vi "IX81 Device Engine.vi"(0 "Unique Notifier Name":string, 11 "COM Port":string[](array[string])) -> ()   [LabVIEW 2020]
uses:
  Microscopes Type Defs/Microscope Notifier.ctl
  Microscopes Type Defs/Microscope Actions.ctl
  <vilib>/Instr/_visa.llb/VISA Configure Serial Port (Instr).vi
panel:
  out "Objective Z Position (um)":dbl
  in  "Lock Base":bool
  out "Last Error":errorcluster
  in  "Quit":bool
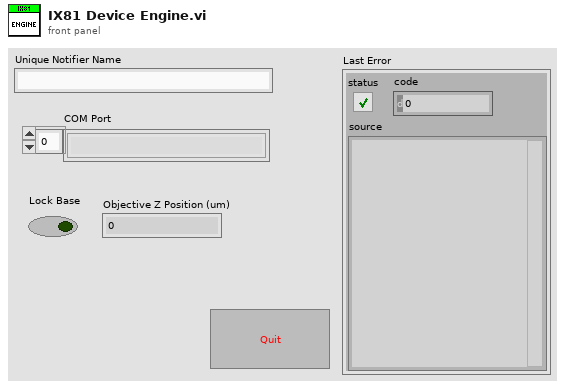
[diagram p1: front panel]
types:
  T1 = typedef "Microscope Actions.ctl" = enum16{"Do Nothing", "Lock Base", "Get Objective Index", "Get Objective Z Position", "Get Lamp State", "Get Lamp Power", "Get Output Port", "Get Shutter State", "Get Dichroic Wheel Position", "Set Lamp Index", "Set Shutter Index", "Set Objective Z Position", "Set Lamp State", "Set Lamp Power", "Set Output Port", "Set Shutter State", "Set Dichroic Wheel Position", "Set Objective", "Abort Move", "Set Parameter", "Get Parameter", "Quit"}
  T2 = typedef "Microscope Notifier.ctl" = cluster{"Actions":T1, "Action Done":bool, "Objective Index":u8, "Objective Z Position (um)":dbl, "Lamp Index":u8, "Lamp State":bool, "Output Port":u8, "Shutter Index":u8, "Shutter State":bool, "Dichroic Wheel Position":u8, "Parameter":string, "Parameter Value":string, "Base Locked?":bool, "Obj Speed":u32, "Obj Acceleration":u32, "Obj Deceleration":u32, "Lamp Power (%)":dbl}
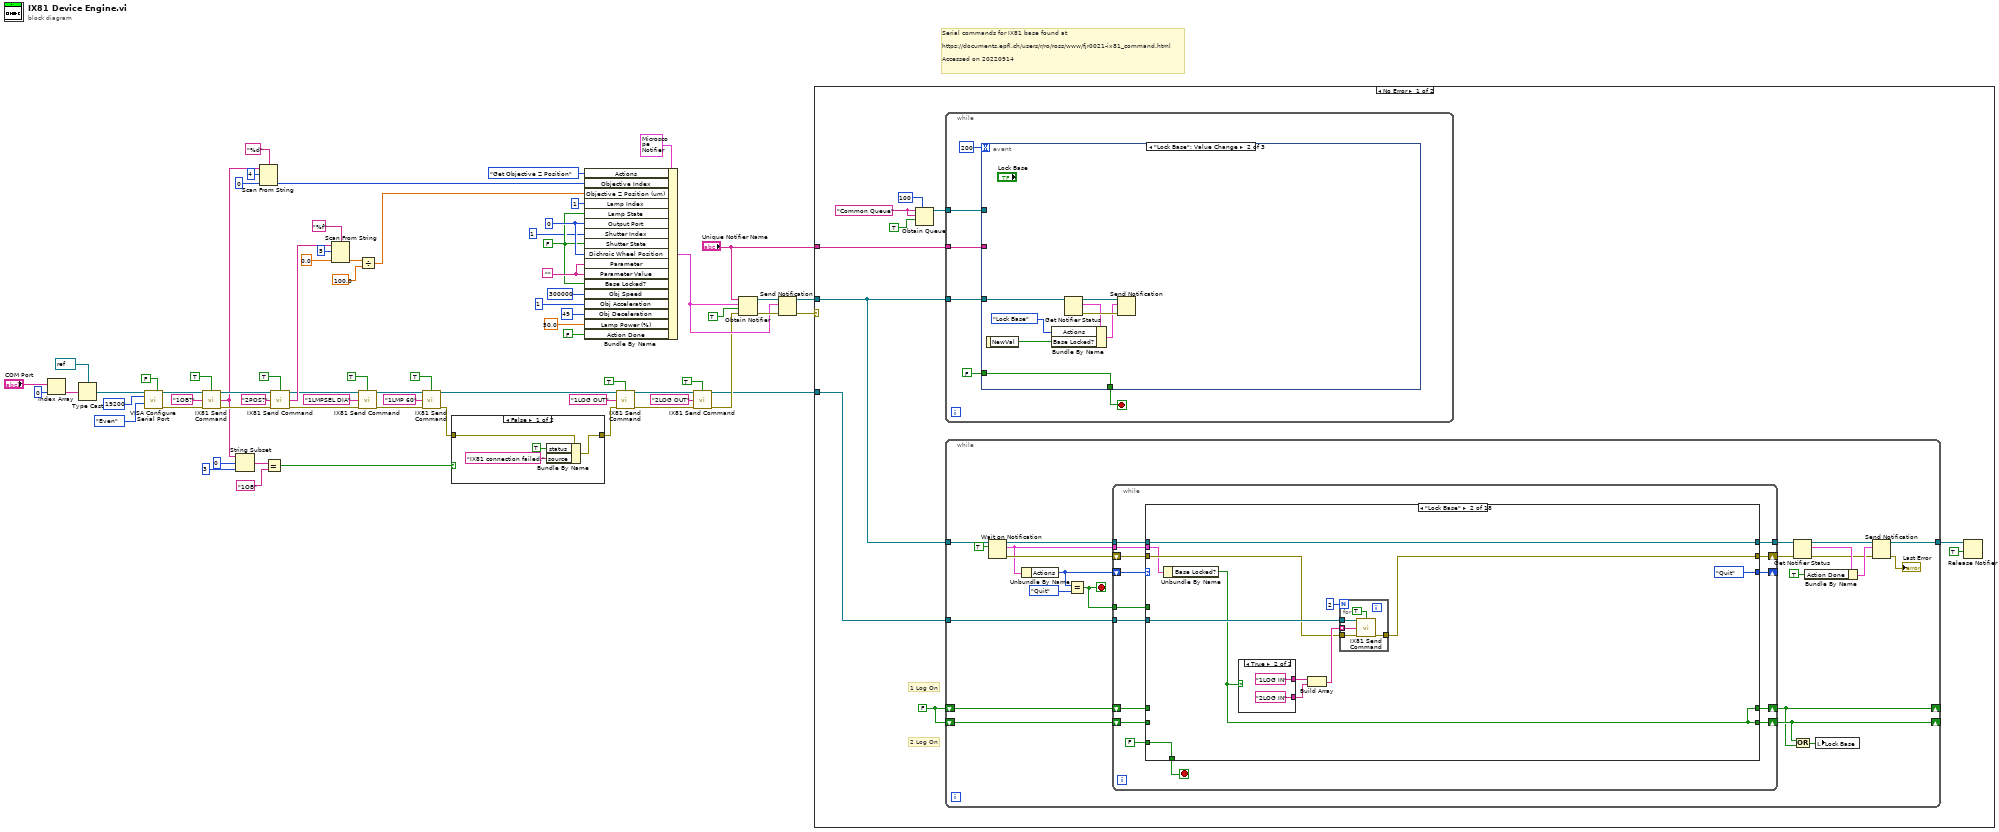
[diagram p0: block diagram]
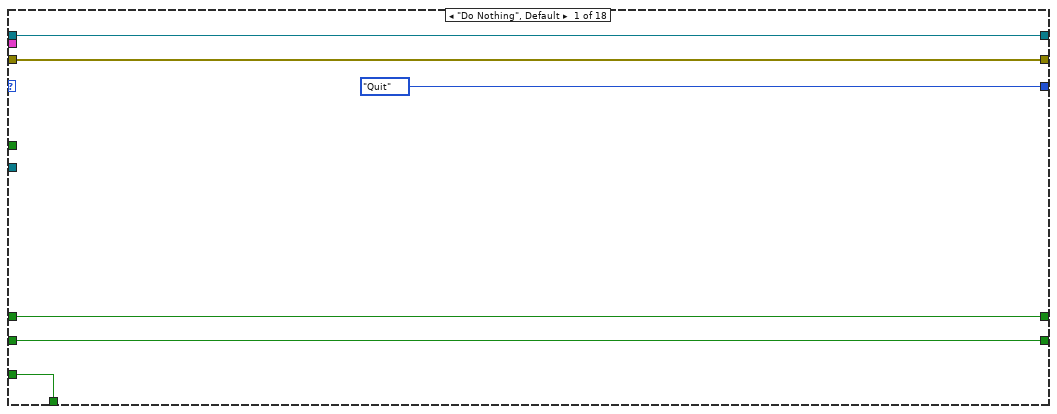
[diagram p2: hidden frame]
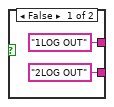
[diagram p3: hidden frame]
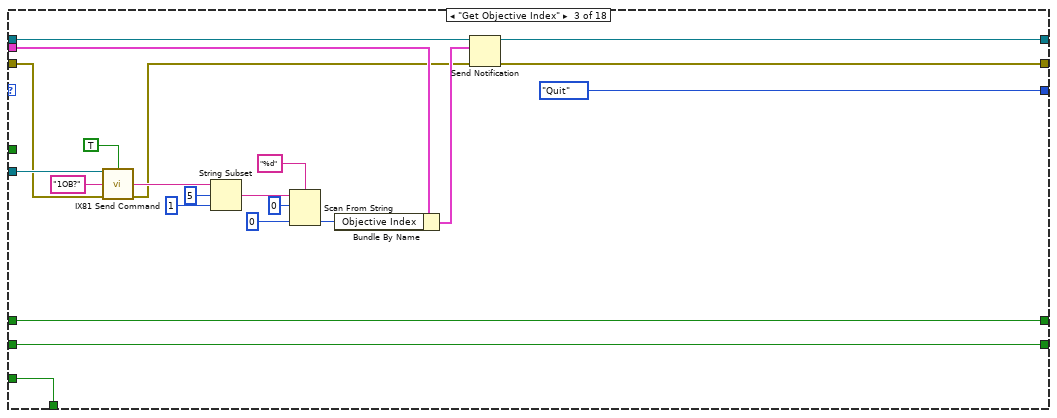
[diagram p4: hidden frame]
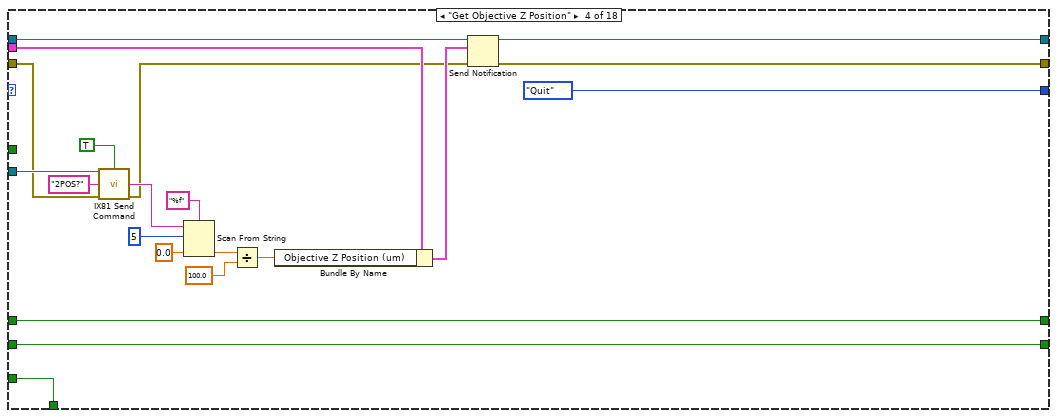
[diagram p5: hidden frame]
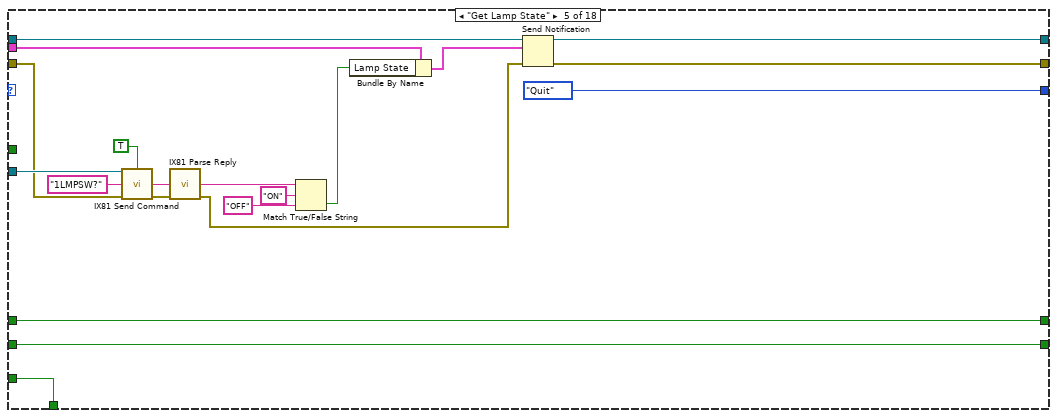
[diagram p6: hidden frame]
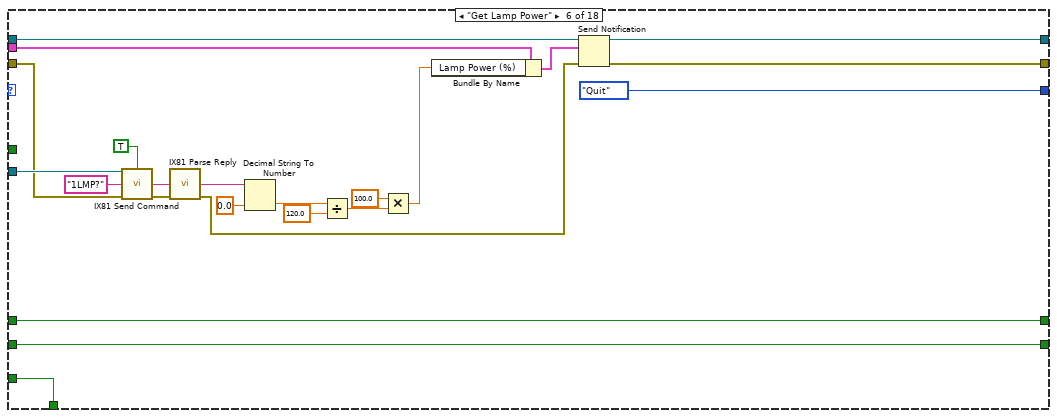
[diagram p7: hidden frame]
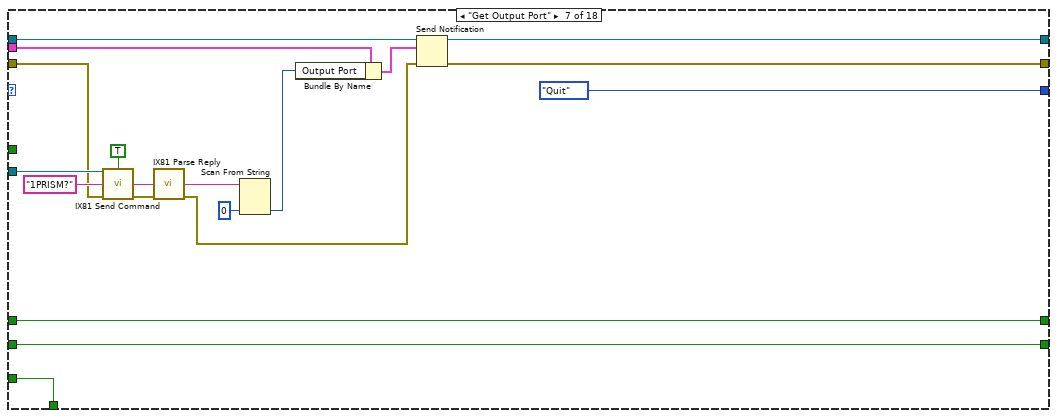
[diagram p8: hidden frame]
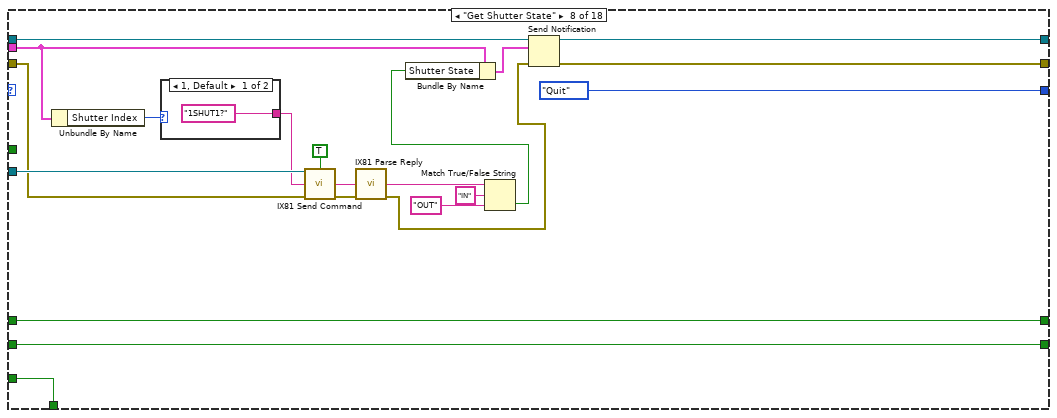
[diagram p9: hidden frame]
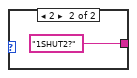
[diagram p10: hidden frame]
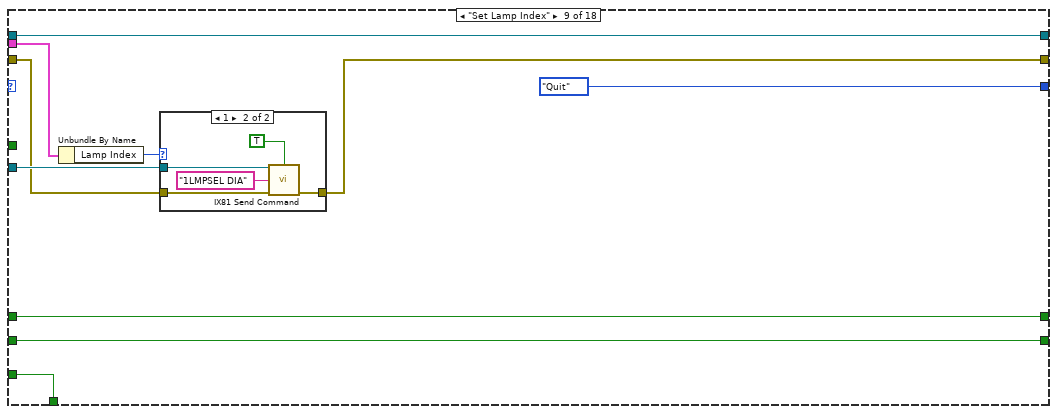
[diagram p11: hidden frame]
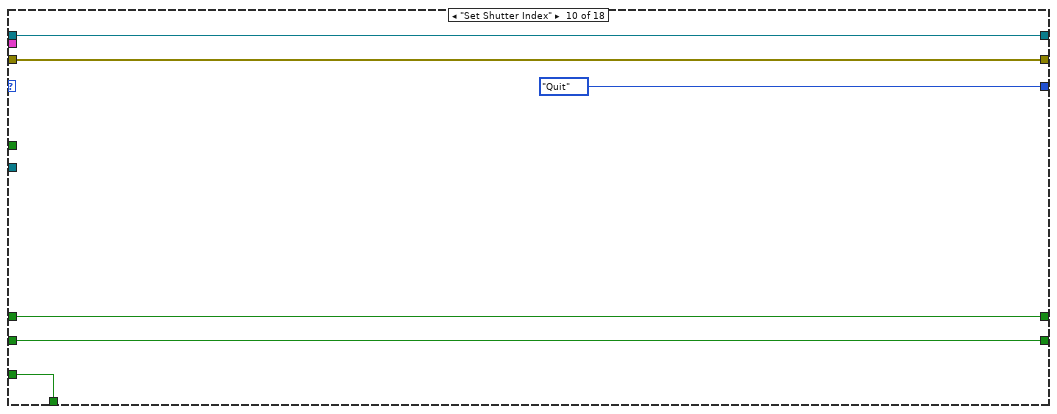
[diagram p13: hidden frame]
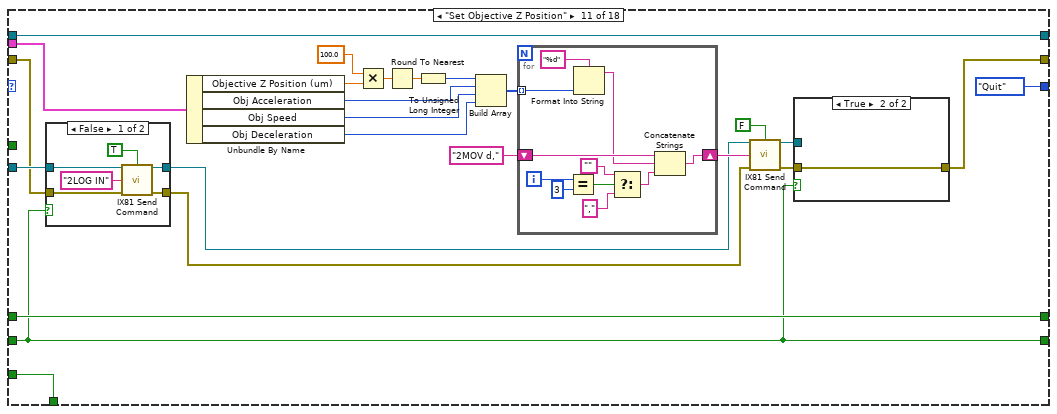
[diagram p14: hidden frame]
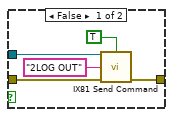
[diagram p15: hidden frame]
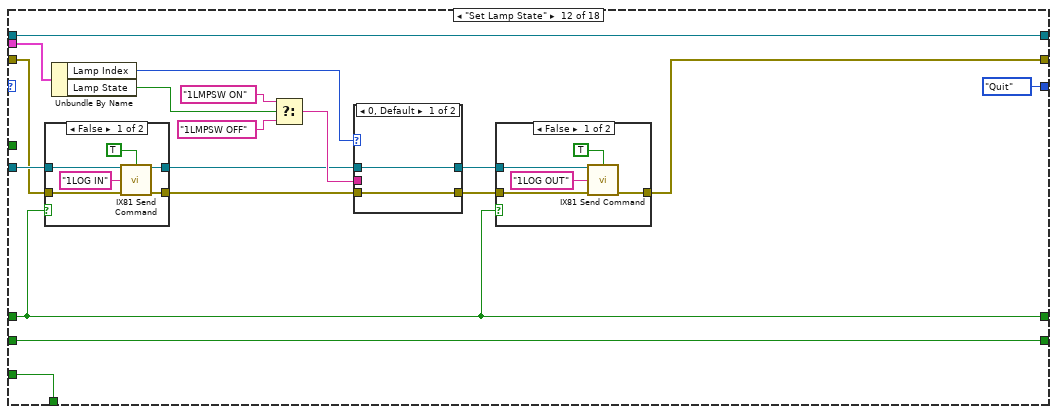
[diagram p17: hidden frame]
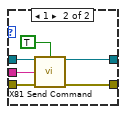
[diagram p19: hidden frame]
diagram:
  w23 = FALSE ("Shutter State")
  w50 = ""
  w34 = u8 0 ("Lamp Index")
  # "Serial commands for IX81 base found at\n\nhttps://documents.epfl.ch/users/r/ro/ross/www/fjr0021-ix81_command.html\n\nAccessed on 20220914"
  n1 = Index Array(array="COM Port", index=0) -> (element=w69:string)
  n2 = Type Cast(type=refnum<visa-resource-name> refnum ("VISA resource name"), x=w69) -> (*(type *) &x=w57:refnum<visa-resource-name>)
  n3 = call-poly "VISA Configure Serial Port"("VISA resource name"=w57, "Enable Termination\nChar (T)"=FALSE ("Enable Termination\nChar (T)"), "baud rate (9600)"=u32 19200, "parity (0:none)"=enum16{"None", "Odd", "Even", "Mark", "Space"}."Even") -> ("VISA resource name out"=w64:refnum<visa-resource-name>, "error out"=w65:errorcluster)  [unwired: 10 in]
  n4 = call "IX81 Send Command.vi"("VISA Ref"=w64, "Wait for Reply (T)"=TRUE, "Command"="1OB?", "Error In"=w65) -> ("VISA Ref Dup"=w44:refnum<visa-resource-name>, "Reply"=w18:string, "Error Out"=w42:errorcluster)  [unwired: 8 in, 1 out]
  n5 = String Subset(string=w18, offset (0)=0, length (rest)=3 ("length (rest)")) -> (substring=w60:string)
  n6 = Scan From String(format string="%d", input string=w18, initial scan location=u32 4, default 1=u8 0 ("default value 1")) -> (output 1=w19:u8)  [unwired: 1 in, 3 out]
  n7 = Equal?(x=w60, y="1OB") -> (x = y?=w55:bool)
  n8 = call "IX81 Send Command.vi"("VISA Ref"=w44, "Wait for Reply (T)"=TRUE, "Command"="2POS?", "Error In"=w42) -> ("VISA Ref Dup"=w15:refnum<visa-resource-name>, "Reply"=w38:string, "Error Out"=w16:errorcluster)  [unwired: 8 in, 1 out]
  n9 = Scan From String(format string="%f", input string=w38, initial scan location=u32 5, default 1=0.0 ("default value 1")) -> (output 1=w37:dbl)  [unwired: 1 in, 3 out]
  n10 = call "IX81 Send Command.vi"("VISA Ref"=w15, "Wait for Reply (T)"=TRUE, "Command"="1LMPSEL DIA", "Error In"=w16) -> ("VISA Ref Dup"=w10:refnum<visa-resource-name>, "Error Out"=w9:errorcluster)  [unwired: 8 in, 2 out]
  n11 = Divide(x=w37, y=100.0) -> (x/y=w35:dbl)
  n12 = call "IX81 Send Command.vi"("VISA Ref"=w10, "Wait for Reply (T)"=TRUE, "Command"="1LMP 60", "Error In"=w9) -> ("VISA Ref Dup"=w7:refnum<visa-resource-name>, "Error Out"=w8:errorcluster)  [unwired: 8 in, 2 out]
  n13 = case shown="False" w55 {
    tunnel: w8 -> [w75 w76]
    tunnel: [w72 w76] -> w26
    frame False {
      n14 = Bundle By Name(cluster=w75, "status"=TRUE, "source"="IX81 connection failed.") -> (w72:errorcluster)
    }
    frame True {
    }
  }
  n15 = Bundle By Name(cluster=T2 {"Actions"=enum."Get Objective Index", "Action Done"=FALSE, "Objective Index"=0, "Objective Z Position (um)"=0.0, "Lamp Index"=0, "Lamp State"=FALSE, "Output Port"=0, "Shutter Index"=0, "Shutter State"=FALSE, "Dichroic Wheel Position"=0, "Parameter"="", "Parameter Value"="", "Base Locked?"=FALSE, "Obj Speed"=0, "Obj Acceleration"=0, "Obj Deceleration"=0, "Lamp Power (%)"=0.0} ("Microscope Notifier"), "Actions"=Microscope_Actions."Get Objective Z Position", "Objective Index"=w19, "Objective Z Position (um)"=w35, "Lamp Index"=u8 1, "Lamp State"=w23, "Output Port"=w34, "Shutter Index"=u8 1, "Shutter State"=w23, "Dichroic Wheel Position"=w34, "Parameter"=w50, "Parameter Value"=w50, "Base Locked?"=w23, "Obj Speed"=u32 300000, "Obj Acceleration"=u32 1, "Obj Deceleration"=u32 49, "Lamp Power (%)"=50.0, "Action Done"=FALSE) -> (w45:T2)
  n16 = call "IX81 Send Command.vi"("VISA Ref"=w7, "Wait for Reply (T)"=TRUE, "Command"="1LOG OUT", "Error In"=w26) -> ("VISA Ref Dup"=w27:refnum<visa-resource-name>, "Error Out"=w28:errorcluster)  [unwired: 8 in, 2 out]
  n17 = call "IX81 Send Command.vi"("VISA Ref"=w27, "Wait for Reply (T)"=TRUE, "Command"="2LOG OUT", "Error In"=w28) -> ("VISA Ref Dup"=w24:refnum<visa-resource-name>, "Error Out"=w25:errorcluster)  [unwired: 8 in, 2 out]
  n18 = Obtain Notifier(name (unnamed)="Unique Notifier Name", notification data type=w45, create if not found? (T)=TRUE, error in (no error)=w25) -> (notifier out=w49:refnum<notifier>, error out=w47:errorcluster)  [unwired: 1 out]
  n19 = Send Notification(notification=w45, notifier=w49, error in (no error)=w47) -> (notifier out=w48:refnum<notifier>, error out=w46:errorcluster)
  n20 = case shown="No Error" w46 {
    tunnel: "Unique Notifier Name" -> [w82 _]
    tunnel: w48 -> [w77 _]
    tunnel: w24 -> [w79 _]
    frame No Error {
      w78 = FALSE
      w86 = "Common Queue" ("Unique Notifier Name")
      # "2 Log On"
      # "1 Log On"
      n21 = Obtain Queue(max queue size (-1, unlimited)=100, name (unnamed)=w86, element data type=w86, create if not found? (T)=TRUE) -> (queue out=w83:refnum<queue>)  [unwired: 1 in, 2 out]
      n22 = while {
        tunnel: w77 -> [w564]
        tunnel: w83 -> [w561]
        tunnel: w82 -> [w560]
        stop <- w562 stop-if-true
        n23 = event shown="[1] \"Lock Base\": Value Change" {
          selector: _ -> [_ _ _]
          dyn-events: _ -> [_ _ _]
          timeout: 200 -> [_ _ _]
          tunnel: w564 -> [w577 w581 w590]
          tunnel: [w575 w586 TRUE ("status")] -> w562
          tunnel: w561 -> [w571 _ _]
          tunnel: w560 -> [w570 _ _]
          tunnel: FALSE ("status") -> [_ w586 _]
          event Timeout {
            n24 = event-data() -> ()  [unwired: 1 in, 1 out]
            n25 = Get Notifier Status(notifier=w577) -> (notifier out=w567:refnum<notifier>, current notification=w569:T2, error out=w576:errorcluster)  [unwired: 1 in, 2 out]
            n26 = call "Common Device Queue Get Command.vi"("Common Queue"=w571, "Notifier Name"=w570) -> ("Command"=w573:string)  [unwired: 12 in, 1 out]
            n27 = Unbundle By Name(w576) -> ("status"=w575:bool)
            n28 = control-ref of="This VI"() -> (w572:refnum<vi>)
            n29 = call "Common Device Queue Execute Command.vi"("Common Command"=w573, "VI Refnum"=w572) -> ("Quit?"=w574:bool)  [unwired: 12 in, 1 out]
            n30 = case shown="False" w574 {
              selector: w574 -> [_ w578]
              frame False {
              }
              frame True {
                n31 = property on="Quit" class="Bool"("Val(Sgnl)"=w578) -> ()  [unwired: 2 in, 2 out]
              }
            }
            n32 = Bundle By Name(cluster=w569, "Actions"=Microscope_Actions."Get Objective Z Position") -> (w566:T2)
            n33 = Send Notification(notification=w566, notifier=w567) -> ()  [unwired: 1 in, 2 out]
            n34 = Unbundle By Name(w566) -> ("Objective Z Position (um)"=→"Objective Z Position (um)":dbl)
          }
          event "Lock Base": Value Change {
            n35 = event-data() -> ("NewVal"=w579:bool)  [unwired: 1 in]
            n36 = Get Notifier Status(notifier=w581) -> (notifier out=w584:refnum<notifier>, current notification=w583:T2, error out=w585:errorcluster)  [unwired: 1 in, 2 out]
            n37 = Bundle By Name(cluster=w583, "Actions"=Microscope_Actions."Lock Base", "Base Locked?"=w579) -> (w582:T2)
            n38 = Send Notification(notification=w582, notifier=w584, error in (no error)=w585) -> ()  [unwired: 2 out]
          }
          event "Quit": Value Change {
            n39 = event-data() -> ()  [unwired: 1 in, 1 out]
            n40 = for {
              N: 5000 -> [_]
              tunnel: w590 -> [w599]
              tunnel: [w596] -> w587
              tunnel: [w594] -> w588
              stop <- w597 stop-if-true
              n41 = Get Notifier Status(notifier=w599) -> (notifier out=w596:refnum<notifier>, current notification=w594:T2, # waiting=w598:i32)  [unwired: 1 in, 2 out]
              n42 = Greater Than 0?(x=w598) -> (x > 0?=w597:bool)
              n43 = Wait (ms)(milliseconds to wait=u32 1) -> ()  [unwired: 1 out]
            }
            n44 = Bundle By Name(cluster=w588, "Actions"=Microscope_Actions."Quit") -> (w591:T2)
            n45 = Send Notification(notification=w591, notifier=w587) -> ()  [unwired: 1 in, 2 out]
          }
        }
      }
      n46 = while {
        tunnel: w77 -> [w109]
        tunnel: [w95] -> w81
        tunnel: w79 -> [w106]
        shift-right: [w100] -> _
        shift-left: w78 -> [w104]
        shift-right: [w101] -> _
        shift-left: w78 -> [w103]
        stop <- w102 stop-if-true
        n47 = Wait on Notification(notifier=w109, ignore previous (F)=TRUE) -> (notifier out=w89:refnum<notifier>, notification=w105:T2, error out=w107:errorcluster)  [unwired: 2 in, 1 out]
        n48 = Unbundle By Name(w105) -> ("Actions"=w87:T1)
        n49 = Equal?(x=w87, y=Microscope_Actions."Quit") -> (x = y?=w102:bool)
        n50 = while {
          shift-right: [w121] -> _
          shift-left: w87 -> [w122]
          tunnel: w89 -> [w119]
          tunnel: [w118] -> w98
          tunnel: w106 -> [w117]
          tunnel: w105 -> [w116]
          shift-right: [w112] -> w100
          shift-left: w104 -> [w114]
          shift-right: [w111] -> w101
          shift-left: w103 -> [w113]
          tunnel: w102 -> [w110]
          shift-right: [w115] -> w97
          shift-left: w107 -> [w120]
          stop <- w123 stop-if-true
          n51 = case shown="\"Lock Base\"" w122 {
            tunnel: FALSE -> [w129 w142 w173 w194 w214 w237 w256 w277 w289 w301 w326 w369 w412 w444 w481 w513 w537 _]
            tunnel: [w129 w142 w173 w194 w214 w237 w256 w277 w289 w301 w326 w369 w412 w444 w481 w513 w537 TRUE] -> w123
            tunnel: [Microscope_Actions."Quit" ("y") Microscope_Actions."Quit" ("y") Microscope_Actions."Quit" ("y") Microscope_Actions."Quit" ("y") Microscope_Actions."Quit" ("y") Microscope_Actions."Quit" ("y") Microscope_Actions."Quit" ("y") Microscope_Actions."Quit" ("y") Microscope_Actions."Quit" ("y") Microscope_Actions."Quit" ("y") Microscope_Actions."Quit" ("y") Microscope_Actions."Quit" ("y") Microscope_Actions."Quit" ("y") Microscope_Actions."Quit" ("y") Microscope_Actions."Quit" ("y") Microscope_Actions."Quit" ("y") Microscope_Actions."Quit" ("y") Microscope_Actions."Quit" ("y")] -> w121
            tunnel: w120 -> [w127 w135 w162 w185 w202 w225 w250 w272 w282 w297 w318 w365 w408 w440 w477 w510 w529 w541]
            tunnel: w119 -> [w128 w132 w158 w183 w210 w233 w243 w268 w281 w298 w325 w364 w407 w439 w476 w509 w534 w545]
            tunnel: [w128 w132 w157 w182 w209 w232 w242 w267 w281 w298 w325 w364 w407 w439 w476 w509 w534 w545] -> w118
            tunnel: w117 -> [_ w138 w163 w186 w205 w228 w252 w273 w284 _ w319 w366 w409 w441 w478 w511 w532 w542]
            tunnel: w116 -> [_ w134 w160 w179 w207 w230 w244 w263 w285 _ w322 w363 w406 w438 w475 w505 _ _]
            tunnel: [w127 w131 w154 w181 w208 w231 w240 w265 w280 w297 w302 w352 w404 w432 w469 w497 w528 w540] -> w115
            tunnel: w114 -> [w126 _ w153 w175 w212 w235 w254 w275 w288 w300 w323 w353 w405 w433 w470 w512 w536 w538]
            tunnel: w113 -> [w125 _ w152 w174 w211 w234 w253 w274 w287 w299 w303 w368 w411 w443 w480 w498 w535 w539]
            tunnel: [w126 w133 w153 w175 w212 w235 w254 w275 w288 w300 w323 w353 w405 w433 w470 w512 w536 w538] -> w112
            tunnel: [w125 w133 w152 w174 w211 w234 w253 w274 w287 w299 w303 w368 w411 w443 w480 w498 w535 w539] -> w111
            tunnel: w110 -> [_ _ _ _ _ _ _ _ _ _ _ _ _ _ _ _ _ w543]
            frame "Do Nothing", Default {
            }
            frame "Lock Base" {
              n52 = Unbundle By Name(w134) -> ("Base Locked?"=w133:bool)
              n53 = case shown="True" w133 {
                tunnel: ["1LOG OUT" ("Command") "1LOG IN" ("Command")] -> w140
                tunnel: ["2LOG OUT" ("Command") "2LOG IN" ("Command")] -> w139
                frame False {
                }
                frame True {
                }
              }
              n54 = Build Array(w140, w139) -> (w136:string[])
              n55 = for {
                N: 2 -> [_]
                tunnel: w138 -> [w146]
                tunnel: w136 -> [w145] mode=indexing
                tunnel: w135 -> [w144]
                tunnel: [w143] -> w131
                n56 = call "IX81 Send Command.vi"("VISA Ref"=w146, "Wait for Reply (T)"=TRUE, "Command"=w145, "Error In"=w144) -> ("Error Out"=w143:errorcluster)  [unwired: 8 in, 3 out]
              }
            }
            frame "Get Objective Index" {
              n57 = call "IX81 Send Command.vi"("VISA Ref"=w163, "Wait for Reply (T)"=TRUE, "Command"="1OB?", "Error In"=w162) -> ("Reply"=w172:string, "Error Out"=w155:errorcluster)  [unwired: 8 in, 2 out]
              n58 = String Subset(string=w172, offset (0)=5, length (rest)=1 ("length (rest)")) -> (substring=w171:string)
              n59 = Scan From String(format string="%d", input string=w171, initial scan location=u32 0, default 1=u8 0 ("default value 1")) -> (output 1=w159:u8)  [unwired: 1 in, 3 out]
              n60 = Bundle By Name(cluster=w160, "Objective Index"=w159) -> (w156:T2)
              n61 = Send Notification(notification=w156, notifier=w158, error in (no error)=w155) -> (notifier out=w157:refnum<notifier>, error out=w154:errorcluster)
            }
            frame "Get Objective Z Position" {
              n62 = call "IX81 Send Command.vi"("VISA Ref"=w186, "Wait for Reply (T)"=TRUE, "Command"="2POS?", "Error In"=w185) -> ("Reply"=w184:string, "Error Out"=w176:errorcluster)  [unwired: 8 in, 2 out]
              n63 = Scan From String(format string="%f", input string=w184, initial scan location=u32 5, default 1=0.0 ("default value 1")) -> (output 1=w190:dbl)  [unwired: 1 in, 3 out]
              n64 = Divide(x=w190, y=100.0) -> (x/y=w178:dbl)
              n65 = Bundle By Name(cluster=w179, "Objective Z Position (um)"=w178) -> (w177:T2)
              n66 = Send Notification(notification=w177, notifier=w183, error in (no error)=w176) -> (notifier out=w182:refnum<notifier>, error out=w181:errorcluster)
            }
            frame "Get Lamp State" {
              n67 = call "IX81 Send Command.vi"("VISA Ref"=w205, "Wait for Reply (T)"=TRUE, "Command"="1LMPSW?", "Error In"=w202) -> ("Reply"=w197:string, "Error Out"=w198:errorcluster)  [unwired: 8 in, 2 out]
              n68 = call "IX81 Parse Reply.vi"("Reply In"=w197, "Error In"=w198) -> ("Reply Out"=w199:string, "Error Out"=w196:errorcluster)  [unwired: 12 in]
              n69 = Match True/False String(2:"OFF" ("false string"), 3:"ON" ("true string"), 4:w199) -> (0:w195:bool)  [unwired: 1 out]
              n70 = Bundle By Name(cluster=w207, "Lamp State"=w195) -> (w206:T2)
              n71 = Send Notification(notification=w206, notifier=w210, error in (no error)=w196) -> (notifier out=w209:refnum<notifier>, error out=w208:errorcluster)
            }
            frame "Get Lamp Power" {
              n72 = call "IX81 Send Command.vi"("VISA Ref"=w228, "Wait for Reply (T)"=TRUE, "Command"="1LMP?", "Error In"=w225) -> ("Reply"=w223:string, "Error Out"=w224:errorcluster)  [unwired: 8 in, 2 out]
              n73 = call "IX81 Parse Reply.vi"("Reply In"=w223, "Error In"=w224) -> ("Reply Out"=w222:string, "Error Out"=w215:errorcluster)  [unwired: 12 in]
              n74 = Decimal String To Number(string=w222, default (0L)=0.0 ("default value 1")) -> (number=w220:dbl)  [unwired: 1 in, 1 out]
              n75 = Divide(x=w220, y=120.0) -> (x/y=w218:dbl)
              n76 = Multiply(x=100.0, y=w218) -> (x*y=w216:dbl)
              n77 = Bundle By Name(cluster=w230, "Lamp Power (%)"=w216) -> (w229:T2)
              n78 = Send Notification(notification=w229, notifier=w233, error in (no error)=w215) -> (notifier out=w232:refnum<notifier>, error out=w231:errorcluster)
            }
            frame "Get Output Port" {
              n79 = call "IX81 Send Command.vi"("VISA Ref"=w252, "Wait for Reply (T)"=TRUE, "Command"="1PRISM?", "Error In"=w250) -> ("Reply"=w248:string, "Error Out"=w247:errorcluster)  [unwired: 8 in, 2 out]
              n80 = call "IX81 Parse Reply.vi"("Reply In"=w248, "Error In"=w247) -> ("Reply Out"=w245:string, "Error Out"=w239:errorcluster)  [unwired: 12 in]
              n81 = Scan From String(input string=w245, default 1=u8 0 ("default value 1")) -> (output 1=w238:u8)  [unwired: 3 in, 3 out]
              n82 = Bundle By Name(cluster=w244, "Output Port"=w238) -> (w241:T2)
              n83 = Send Notification(notification=w241, notifier=w243, error in (no error)=w239) -> (notifier out=w242:refnum<notifier>, error out=w240:errorcluster)
            }
            frame "Get Shutter State" {
              n84 = Unbundle By Name(w263) -> ("Shutter Index"=w264:u8)
              n85 = case shown="1, Default" w264 {
                tunnel: ["1SHUT1?" ("Command") "1SHUT2?" ("Command")] -> w262
                frame 1, Default {
                }
                frame 2 {
                }
              }
              n86 = call "IX81 Send Command.vi"("VISA Ref"=w273, "Wait for Reply (T)"=TRUE, "Command"=w262, "Error In"=w272) -> ("Reply"=w270:string, "Error Out"=w269:errorcluster)  [unwired: 8 in, 2 out]
              n87 = call "IX81 Parse Reply.vi"("Reply In"=w270, "Error In"=w269) -> ("Reply Out"=w259:string, "Error Out"=w257:errorcluster)  [unwired: 12 in]
              n88 = Match True/False String(2:"OUT" ("false string"), 3:"IN" ("true string"), 4:w259) -> (0:w258:bool)  [unwired: 1 out]
              n89 = Bundle By Name(cluster=w263, "Shutter State"=w258) -> (w266:T2)
              n90 = Send Notification(notification=w266, notifier=w268, error in (no error)=w257) -> (notifier out=w267:refnum<notifier>, error out=w265:errorcluster)
            }
            frame "Set Lamp Index" {
              n91 = Unbundle By Name(w285) -> ("Lamp Index"=w283:u8)
              n92 = case shown="1" w283 {
                tunnel: w284 -> [_ w293]
                tunnel: w282 -> [w290 w292]
                tunnel: [w290 w291] -> w280
                frame 0, Default {
                }
                frame 1 {
                  n93 = call "IX81 Send Command.vi"("VISA Ref"=w293, "Wait for Reply (T)"=TRUE, "Command"="1LMPSEL DIA", "Error In"=w292) -> ("Error Out"=w291:errorcluster)  [unwired: 8 in, 3 out]
                }
              }
            }
            frame "Set Shutter Index" {
            }
            frame "Set Objective Z Position" {
              n94 = case shown="False" w303 {
                tunnel: w319 -> [w347 w351]
                tunnel: w318 -> [w346 w350]
                tunnel: [w345 w351] -> w307
                tunnel: [w344 w350] -> w306
                frame False {
                  n95 = call "IX81 Send Command.vi"("VISA Ref"=w347, "Wait for Reply (T)"=TRUE, "Command"="2LOG IN", "Error In"=w346) -> ("VISA Ref Dup"=w345:refnum<visa-resource-name>, "Error Out"=w344:errorcluster)  [unwired: 8 in, 2 out]
                }
                frame True {
                }
              }
              n96 = Unbundle By Name(w322) -> ("Objective Z Position (um)"=w321:dbl, "Obj Acceleration"=w314:u32, "Obj Speed"=w313:u32, "Obj Deceleration"=w312:u32)
              n97 = Multiply(x=100.0, y=w321) -> (x*y=w317:dbl)
              n98 = Round To Nearest(number=w317) -> (nearest integer value=w316:dbl)
              n99 = To Unsigned Long Integer(number=w316) -> (unsigned 32bit integer=w315:u32)
              n100 = Build Array(w315, w314, w313, w312) -> (w311:u32[])
              n101 = for {
                tunnel: w311 -> [w342] mode=indexing
                shift-right: [w339] -> w308
                shift-left: "2MOV d," ("Command") -> [w341]
                i -> [w334]
                n102 = Equal?(x=w334, y=3) -> (x = y?=w338:bool)
                n103 = Format Into String(format string="%d", w342) -> (resulting string=w340:string)  [unwired: 2 in, 1 out]
                n104 = Select(t="", s=w338, f="," ("string")) -> (s? t:f=w333:string)
                n105 = Concatenate Strings(w341, w340, w333) -> (w339:string)
              }
              n106 = call "IX81 Send Command.vi"("VISA Ref"=w307, "Wait for Reply (T)"=FALSE, "Command"=w308, "Error In"=w306) -> ("VISA Ref Dup"=w305:refnum<visa-resource-name>, "Error Out"=w304:errorcluster)  [unwired: 8 in, 2 out]
              n107 = case shown="True" w303 {
                tunnel: w305 -> [w329 _]
                tunnel: w304 -> [w328 w332]
                tunnel: [w327 w332] -> w302
                frame False {
                  n108 = call "IX81 Send Command.vi"("VISA Ref"=w329, "Wait for Reply (T)"=TRUE, "Command"="2LOG OUT", "Error In"=w328) -> ("Error Out"=w327:errorcluster)  [unwired: 8 in, 3 out]
                }
                frame True {
                }
              }
            }
            frame "Set Lamp State" {
              n109 = case shown="False" w353 {
                tunnel: w366 -> [w387 w391]
                tunnel: w365 -> [w386 w390]
                tunnel: [w385 w391] -> w356
                tunnel: [w384 w390] -> w357
                frame False {
                  n110 = call "IX81 Send Command.vi"("VISA Ref"=w387, "Wait for Reply (T)"=TRUE, "Command"="1LOG IN", "Error In"=w386) -> ("VISA Ref Dup"=w385:refnum<visa-resource-name>, "Error Out"=w384:errorcluster)  [unwired: 8 in, 2 out]
                }
                frame True {
                }
              }
              n111 = Unbundle By Name(w363) -> ("Lamp Index"=w359:u8, "Lamp State"=w360:bool)
              n112 = Select(t="1LMPSW ON" ("Command"), s=w360, f="1LMPSW OFF" ("Command")) -> (s? t:f=w358:string)
              n113 = case shown="0, Default" w359 {
                tunnel: w358 -> [_ w382]
                tunnel: w357 -> [w377 w381]
                tunnel: w356 -> [w376 w380]
                tunnel: [w377 w379] -> w354
                tunnel: [w376 w378] -> w355
                frame 0, Default {
                }
                frame 1 {
                  n114 = call "IX81 Send Command.vi"("VISA Ref"=w380, "Wait for Reply (T)"=TRUE, "Command"=w382, "Error In"=w381) -> ("VISA Ref Dup"=w378:refnum<visa-resource-name>, "Error Out"=w379:errorcluster)  [unwired: 8 in, 2 out]
                }
              }
              n115 = case shown="False" w353 {
                tunnel: w355 -> [w372 _]
                tunnel: w354 -> [w371 w375]
                tunnel: [w370 w375] -> w352
                frame False {
                  n116 = call "IX81 Send Command.vi"("VISA Ref"=w372, "Wait for Reply (T)"=TRUE, "Command"="1LOG OUT", "Error In"=w371) -> ("Error Out"=w370:errorcluster)  [unwired: 8 in, 3 out]
                }
                frame True {
                }
              }
            }
            frame "Set Lamp Power" {
              n117 = case shown="False" w405 {
                tunnel: w409 -> [w422 w426]
                tunnel: w408 -> [w421 w425]
                tunnel: [w420 w426] -> w396
                tunnel: [w419 w425] -> w395
                frame False {
                  n118 = call "IX81 Send Command.vi"("VISA Ref"=w422, "Wait for Reply (T)"=TRUE, "Command"="1LOG IN", "Error In"=w421) -> ("VISA Ref Dup"=w420:refnum<visa-resource-name>, "Error Out"=w419:errorcluster)  [unwired: 8 in, 2 out]
                }
                frame True {
                }
              }
              n119 = Unbundle By Name(w406) -> ("Lamp Power (%)"=w403:dbl)
              n120 = Divide(x=w403, y=100.0) -> (x/y=w401:dbl)
              n121 = Multiply(x=w401, y=120.0) -> (x*y=w399:dbl)
              n122 = Format Into String(format string="%d", initial string="1LMP " ("Command"), w399) -> (resulting string=w394:string)  [unwired: 1 in, 1 out]
              n123 = call "IX81 Send Command.vi"("VISA Ref"=w396, "Command"=w394, "Error In"=w395) -> ("VISA Ref Dup"=w393:refnum<visa-resource-name>, "Error Out"=w392:errorcluster)  [unwired: 9 in, 2 out]
              n124 = case shown="False" w405 {
                tunnel: w393 -> [w415 _]
                tunnel: w392 -> [w414 w418]
                tunnel: [w413 w418] -> w404
                frame False {
                  n125 = call "IX81 Send Command.vi"("VISA Ref"=w415, "Wait for Reply (T)"=TRUE, "Command"="1LOG OUT", "Error In"=w414) -> ("Error Out"=w413:errorcluster)  [unwired: 8 in, 3 out]
                }
                frame True {
                }
              }
            }
            frame "Set Output Port" {
              n126 = case shown="False" w433 {
                tunnel: w441 -> [w454 w458]
                tunnel: w440 -> [w453 w457]
                tunnel: [w452 w458] -> w436
                tunnel: [w451 w457] -> w437
                frame False {
                  n127 = call "IX81 Send Command.vi"("VISA Ref"=w454, "Wait for Reply (T)"=TRUE, "Command"="1LOG IN", "Error In"=w453) -> ("VISA Ref Dup"=w452:refnum<visa-resource-name>, "Error Out"=w451:errorcluster)  [unwired: 8 in, 2 out]
                }
                frame True {
                }
              }
              n128 = Unbundle By Name(w438) -> ("Output Port"=w430:u8)
              n129 = Format Into String(format string="%d", initial string="1PRISM ", w430) -> (resulting string=w427:string)  [unwired: 1 in, 1 out]
              n130 = call "IX81 Send Command.vi"("VISA Ref"=w436, "Wait for Reply (T)"=TRUE, "Command"=w427, "Error In"=w437) -> ("VISA Ref Dup"=w435:refnum<visa-resource-name>, "Error Out"=w434:errorcluster)  [unwired: 8 in, 2 out]
              n131 = case shown="False" w433 {
                tunnel: w435 -> [w447 _]
                tunnel: w434 -> [w446 w450]
                tunnel: [w445 w450] -> w432
                frame False {
                  n132 = call "IX81 Send Command.vi"("VISA Ref"=w447, "Wait for Reply (T)"=TRUE, "Command"="1LOG OUT", "Error In"=w446) -> ("Error Out"=w445:errorcluster)  [unwired: 8 in, 3 out]
                }
                frame True {
                }
              }
            }
            frame "Set Shutter State" {
              n133 = case shown="False" w470 {
                tunnel: w478 -> [w491 w495]
                tunnel: w477 -> [w490 w494]
                tunnel: [w489 w495] -> w473
                tunnel: [w488 w494] -> w474
                frame False {
                  n134 = call "IX81 Send Command.vi"("VISA Ref"=w491, "Wait for Reply (T)"=TRUE, "Command"="1LOG IN", "Error In"=w490) -> ("VISA Ref Dup"=w489:refnum<visa-resource-name>, "Error Out"=w488:errorcluster)  [unwired: 8 in, 2 out]
                }
                frame True {
                }
              }
              n135 = Unbundle By Name(w475) -> ("Shutter Index"=w465:u8, "Shutter State"=w464:bool)
              n136 = Select(t=" IN" ("initial string"), s=w464, f=" OUT" ("initial string")) -> (s? t:f=w460:string)
              n137 = Format Into String(format string="%d", initial string="1SHUT", w465) -> (resulting string=w461:string)  [unwired: 1 in, 1 out]
              n138 = Concatenate Strings(w461, w460) -> (w459:string)
              n139 = call "IX81 Send Command.vi"("VISA Ref"=w473, "Wait for Reply (T)"=TRUE, "Command"=w459, "Error In"=w474) -> ("VISA Ref Dup"=w472:refnum<visa-resource-name>, "Error Out"=w471:errorcluster)  [unwired: 8 in, 2 out]
              n140 = case shown="False" w470 {
                tunnel: w472 -> [w484 _]
                tunnel: w471 -> [w483 w487]
                tunnel: [w482 w487] -> w469
                frame False {
                  n141 = call "IX81 Send Command.vi"("VISA Ref"=w484, "Wait for Reply (T)"=TRUE, "Command"="1LOG OUT", "Error In"=w483) -> ("Error Out"=w482:errorcluster)  [unwired: 8 in, 3 out]
                }
                frame True {
                }
              }
            }
            frame "Set Objective" {
              n142 = Unbundle By Name(w505) -> ("Objective Index"=w506:u8)
              n143 = case shown="False" w498 {
                tunnel: w511 -> [w523 w527]
                tunnel: w510 -> [w522 w526]
                tunnel: [w521 w527] -> w504
                tunnel: [w520 w526] -> w502
                frame False {
                  n144 = call "IX81 Send Command.vi"("VISA Ref"=w523, "Wait for Reply (T)"=TRUE, "Command"="1LOG IN", "Error In"=w522) -> ("VISA Ref Dup"=w521:refnum<visa-resource-name>, "Error Out"=w520:errorcluster)  [unwired: 8 in, 2 out]
                }
                frame True {
                }
              }
              n145 = Format Into String(format string="%d", initial string="1OB ", w506) -> (resulting string=w503:string)  [unwired: 1 in, 1 out]
              n146 = call "IX81 Send Command.vi"("VISA Ref"=w504, "Wait for Reply (T)"=TRUE, "Command"=w503, "Error In"=w502) -> ("VISA Ref Dup"=w500:refnum<visa-resource-name>, "Error Out"=w499:errorcluster)  [unwired: 8 in, 2 out]
              n147 = case shown="False" w498 {
                tunnel: w500 -> [w516 _]
                tunnel: w499 -> [w515 w519]
                tunnel: [w514 w519] -> w497
                frame False {
                  n148 = call "IX81 Send Command.vi"("VISA Ref"=w516, "Wait for Reply (T)"=TRUE, "Command"="1LOG OUT", "Error In"=w515) -> ("Error Out"=w514:errorcluster)  [unwired: 8 in, 3 out]
                }
                frame True {
                }
              }
            }
            frame "Abort Move" {
              n149 = call "IX81 Send Command.vi"("VISA Ref"=w532, "Wait for Reply (T)"=TRUE, "Command"="2STOP", "Error In"=w529) -> ("Error Out"=w528:errorcluster)  [unwired: 8 in, 3 out]
            }
            frame "Quit" {
              n150 = case shown="False" w543 {
                tunnel: w542 -> [_ w550]
                tunnel: w541 -> [w547 w549]
                tunnel: [w547 w548] -> w540
                frame False {
                }
                frame True {
                  n151 = call "IX81 Send Command.vi"("VISA Ref"=w550, "Wait for Reply (T)"=TRUE, "Command"="1LOG OUT", "Error In"=w549) -> ("VISA Ref Dup"=w558:refnum<visa-resource-name>, "Error Out"=w557:errorcluster)  [unwired: 8 in, 2 out]
                  n152 = call "IX81 Send Command.vi"("VISA Ref"=w558, "Wait for Reply (T)"=TRUE, "Command"="2LOG OUT", "Error In"=w557) -> ("VISA Ref Dup"=w556:refnum<visa-resource-name>, "Error Out"=w555:errorcluster)  [unwired: 8 in, 2 out]
                  n153 = VISA Close(VISA resource name=w556, error in (no error)=w555) -> (error out=w548:errorcluster)
                }
              }
            }
          }
        }
        n154 = Get Notifier Status(notifier=w98, error in (no error)=w97) -> (notifier out=w96:refnum<notifier>, current notification=w94:T2, error out=w90:errorcluster)  [unwired: 2 out]
        n155 = Or(x=w101, y=w100) -> (x .or. y?=w99:bool)
        n156 = Bundle By Name(cluster=w94, "Action Done"=TRUE) -> (w92:T2)
        n157 = local write "Lock Base"(w99) -> ()
        n158 = Send Notification(notification=w92, notifier=w96, error in (no error)=w90) -> (notifier out=w95:refnum<notifier>, error out=→"Last Error":errorcluster)
      }
      n159 = Release Notifier(notifier=w81, force destroy? (F)=TRUE) -> ()  [unwired: 1 in, 3 out]
    }
    frame Error {
    }
  }
